vi "GetLCDResultValue.vi"(8 "error in (no error)":errorcluster, 11 "Analysis_LCD_Parameter":T2={"ROI"={"Global Rectangle"=[27, 55, 270, 147], "Contours"=[{"Contour Type"=0, "ROI Type"=3, "Points"=[27, 55, 270, 147]}]}, "Number of Matches Requested"=1} {"Number of Matches Requested" min=1 max=9999}) -> (0 "error out":errorcluster, 3 "ResultValues":string[](array[string]))   [LabVIEW 2015]
uses:
  Controls/LCD/Analysis_LCD_Parameter.ctl
panel:
  in  "data":T1
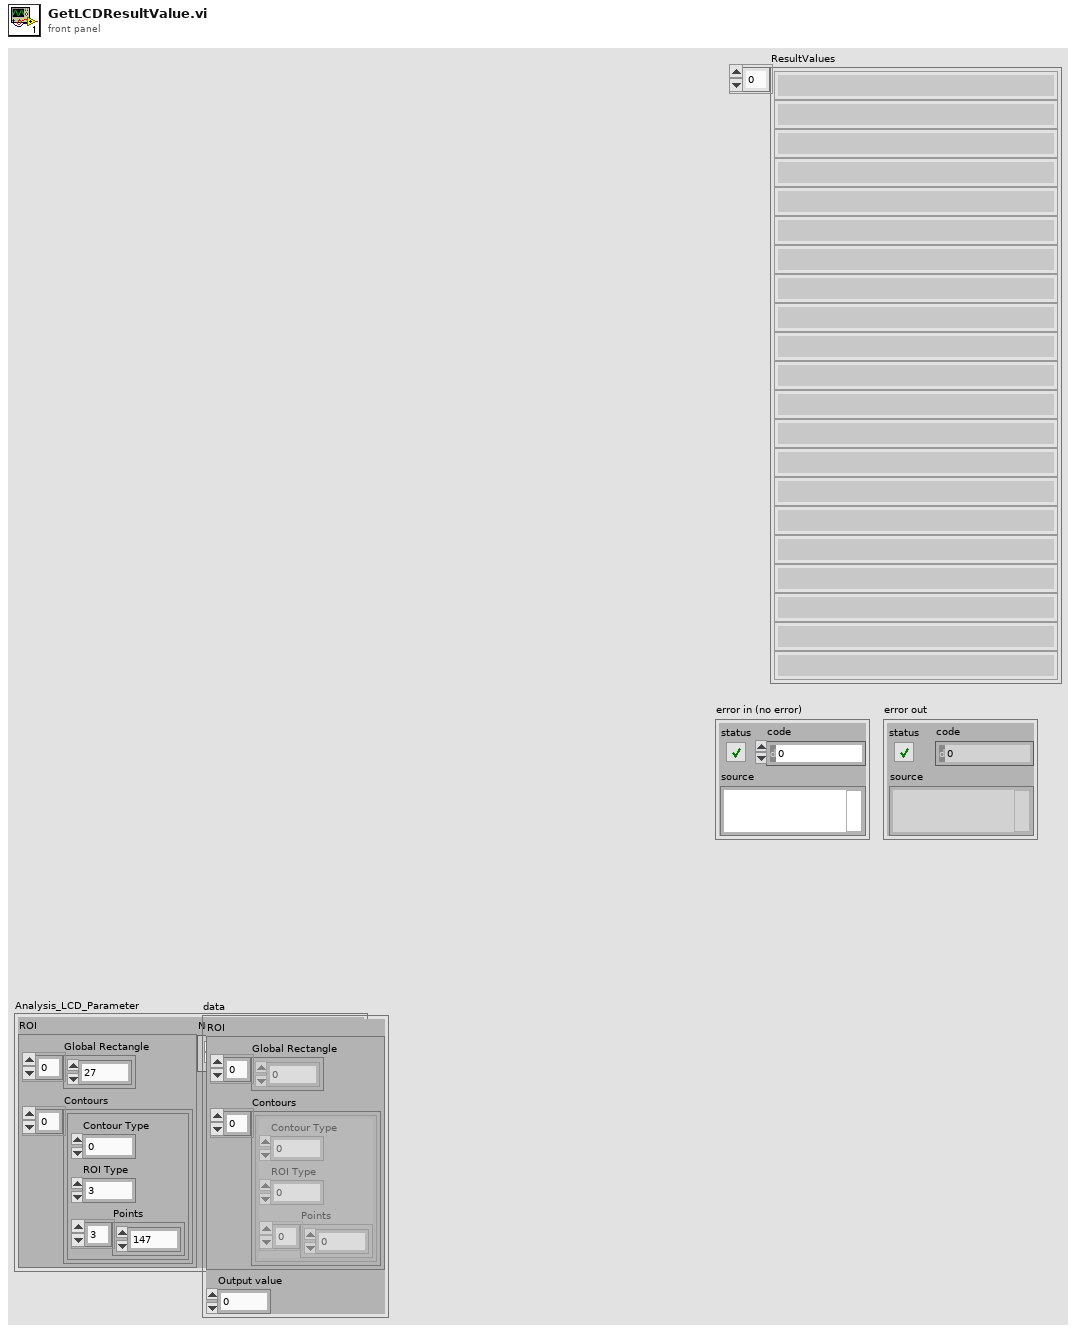
[diagram p1: front panel]
types:
  T1 = cluster{"ROI":cluster{"Global Rectangle":i32[], "Contours":cluster{"Contour Type":u32, "ROI Type":u32, "Points":i32[]}[]}, "Output value":dbl}
  T2 = typedef "Analysis_LCD_Parameter.ctl" = cluster{"ROI":cluster{"Global Rectangle":i32[], "Contours":cluster{"Contour Type":u32, "ROI Type":u32, "Points":i32[]}[]}, "Number of Matches Requested":i32}
  T3 = cluster{"Global Rectangle":i32[], "Contours":cluster{"Contour Type":u32, "ROI Type":u32, "Points":i32[]}[]}
  T4 = cluster{"Contour Type":u32, "ROI Type":u32, "Points":i32[]}[]
  T5 = cluster{"Contour Type":u32, "ROI Type":u32, "Points":i32[]}
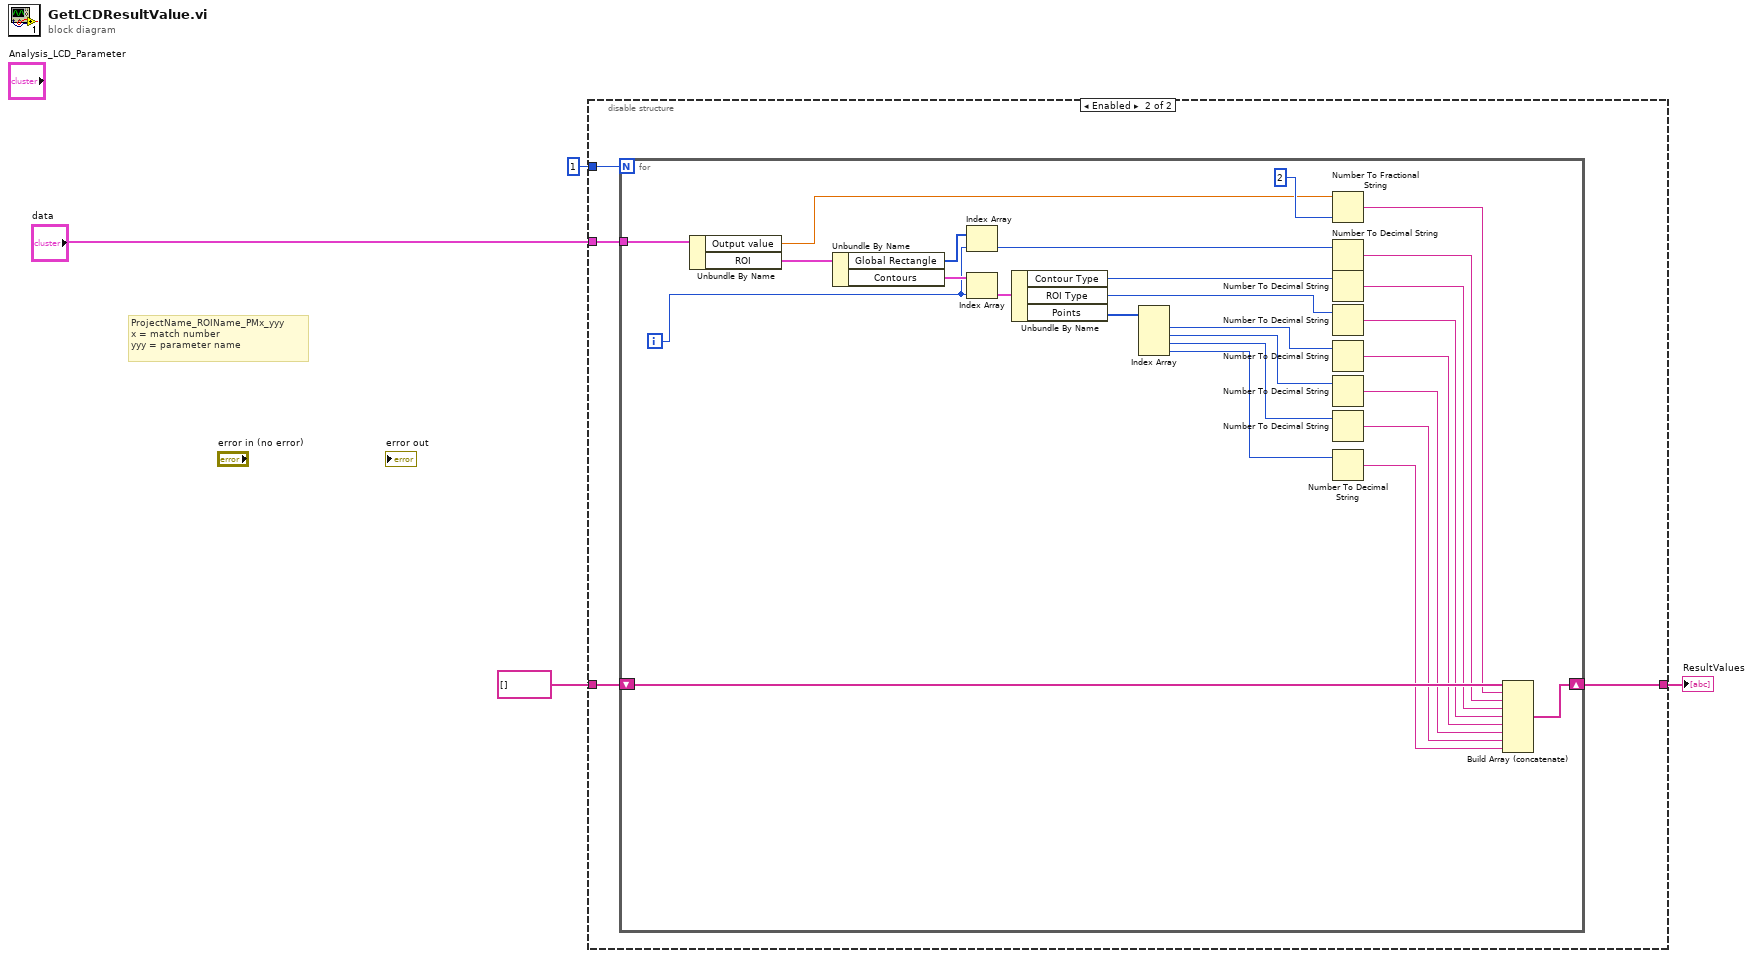
[diagram p0: block diagram]
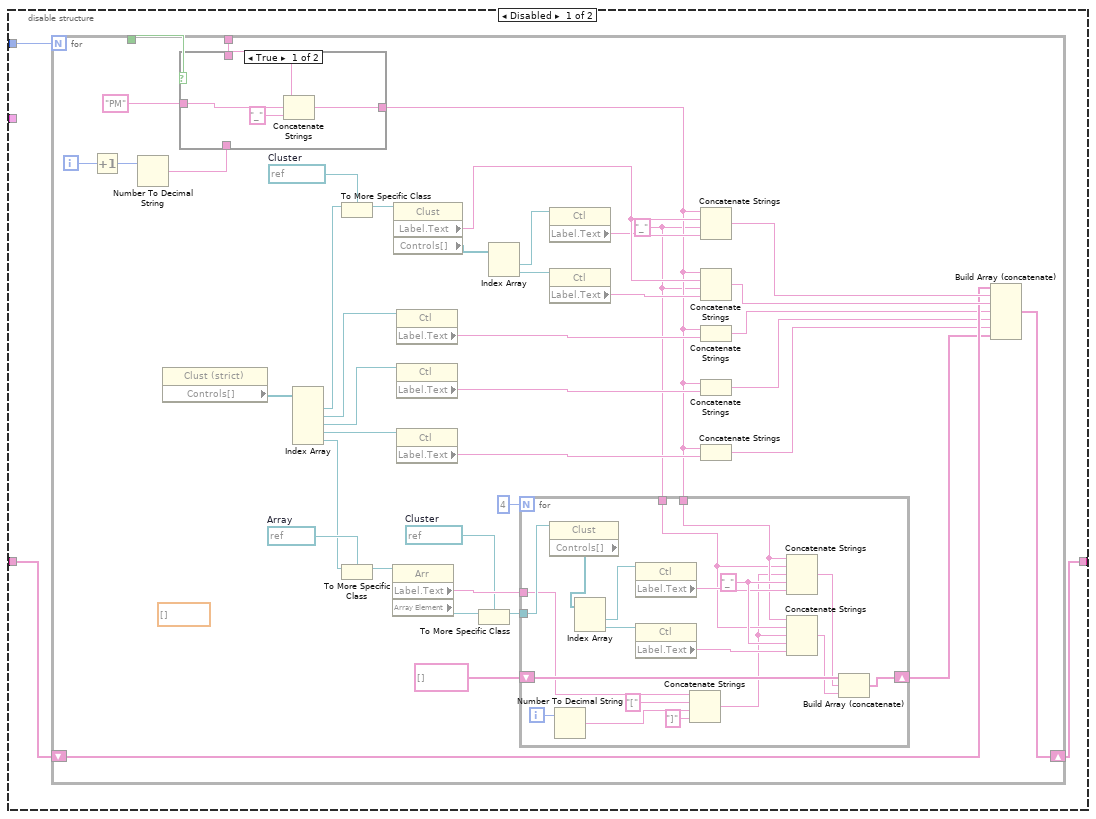
[diagram p2: hidden frame]
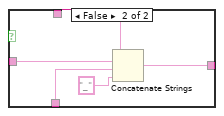
[diagram p3: hidden frame]
diagram:
  # "ProjectName_ROIName_PMx_yyy\nx = match number\nyyy = parameter name"
  n1 = disable-structure shown="Enabled" {
    disable-tunnel: 1 ("Number of Matches Requested") -> [w8 w82]
    disable-tunnel: string[] [] -> [w7 w81]
    disable-tunnel: [w6 w80] -> w3
    disable-tunnel: "data" -> [_ w79]
    frame Disabled {
      n2 = for {
        N: w8 -> [_]
        tunnel: _ -> [w30]
        shift-right: [w32] -> w6
        shift-left: w7 -> [w33]
        tunnel: [w31] -> w5
        i -> [w36]
        w15 = refnum<vi> refnum  # Cluster
        (unwired) dbl[] []
        w20 = refnum<vi> refnum  # Array
        w11 = "_" ("string")
        w46 = refnum<vi> refnum  # Cluster
        n3 = Increment(x=w36) -> (x+1=w35:i32)
        n4 = Number To Decimal String(number=w35) -> (decimal integer string=w29:string)  [unwired: 1 in]
        n5 = property class="Clust (strict)"() -> (reference=w50:refnum<vi>, "Controls[]"=w49:refnum<vi>[])  [unwired: 1 in, 2 out]
        n6 = case shown="True" w31 {
          tunnel: w30 -> [w73 w78]
          tunnel: w29 -> [_ w75]
          tunnel: [w72 w77] -> w12
          tunnel: "PM" ("string") -> [w71 w74]
          frame True {
            n7 = Concatenate Strings(w73, w71, "_" ("string")) -> (w72:string)
          }
          frame False {
            n8 = Concatenate Strings(w78, w74, w75, "_" ("string")) -> (w77:string)
          }
        }
        n9 = Index Array(array=w49) -> (element #1=w48:refnum<vi>, element #2=w27:refnum<vi>, element #3=w26:refnum<vi>, element #4=w39:refnum<vi>, element #5=w19:refnum<vi>)  [unwired: 5 in]
        n10 = To More Specific Class(target class=w46, reference=w48) -> (specific class reference=w47:refnum<vi>)  [unwired: 1 in, 1 out]
        n11 = To More Specific Class(target class=w20, reference=w19) -> (specific class reference=w18:refnum<vi>)  [unwired: 1 in, 1 out]
        n12 = property class="Arr"(reference=w18) -> ("Label.Text"=w17:string, "Array Element"=w14:refnum<vi>)  [unwired: 1 in, 2 out]
        n13 = property class="Clust"(reference=w47) -> ("Label.Text"=w42:string, "Controls[]"=w45:refnum<vi>[])  [unwired: 1 in, 2 out]
        n14 = property class="Ctl"(reference=w27) -> ("Label.Text"=w25:string)  [unwired: 1 in, 2 out]
        n15 = property class="Ctl"(reference=w26) -> ("Label.Text"=w24:string)  [unwired: 1 in, 2 out]
        n16 = property class="Ctl"(reference=w39) -> ("Label.Text"=w34:string)  [unwired: 1 in, 2 out]
        n17 = To More Specific Class(target class=w15, reference=w14) -> (specific class reference=w13:refnum<vi>)  [unwired: 1 in, 1 out]
        n18 = Index Array(array=w45) -> (element #1=w44:refnum<vi>, element #2=w43:refnum<vi>)  [unwired: 2 in]
        n19 = for {
          N: 4 -> [_]
          tunnel: w17 -> [w55]
          tunnel: w13 -> [w69]
          tunnel: w12 -> [w62]
          tunnel: w11 -> [w61]
          shift-right: [w57] -> w9
          shift-left: string[] [] -> [w60]
          i -> [w56]
          w68 = "_" ("string")
          n20 = property class="Clust"(reference=w69) -> ("Controls[]"=w63:refnum<vi>[])  [unwired: 1 in, 2 out]
          n21 = Number To Decimal String(number=w56) -> (decimal integer string=w53:string)  [unwired: 1 in]
          n22 = Index Array(array=w63) -> (element #1=w64:refnum<vi>, element #2=w65:refnum<vi>)  [unwired: 2 in]
          n23 = property class="Ctl"(reference=w64) -> ("Label.Text"=w66:string)  [unwired: 1 in, 2 out]
          n24 = property class="Ctl"(reference=w65) -> ("Label.Text"=w67:string)  [unwired: 1 in, 2 out]
          n25 = Concatenate Strings(w55, "[" ("string"), w53, "]" ("string")) -> (w51:string)
          n26 = Concatenate Strings(w62, w61, w51, w68, w66) -> (w59:string)
          n27 = Concatenate Strings(w62, w61, w51, w68, w67) -> (w58:string)
          n28 = Build Array (concatenate)(w60, w59, w58) -> (w57:string[])
        }
        n29 = property class="Ctl"(reference=w44) -> ("Label.Text"=w41:string)  [unwired: 1 in, 2 out]
        n30 = property class="Ctl"(reference=w43) -> ("Label.Text"=w40:string)  [unwired: 1 in, 2 out]
        n31 = Concatenate Strings(w12, w42, w11, w41) -> (w38:string)
        n32 = Concatenate Strings(w12, w42, w11, w40) -> (w37:string)
        n33 = Concatenate Strings(w12, w25) -> (w21:string)
        n34 = Concatenate Strings(w12, w24) -> (w22:string)
        n35 = Concatenate Strings(w12, w34) -> (w23:string)
        n36 = Build Array (concatenate)(w33, w38, w37, w21, w22, w23, w9) -> (w32:string[])
      }
    }
    frame Enabled {
      n37 = for {
        N: w82 -> [_]
        shift-right: [w106] -> w80
        shift-left: w81 -> [w107]
        tunnel: w79 -> [w108]
        i -> [w99]
        n38 = Unbundle By Name(w108) -> ("Output value"=w104:dbl, "ROI"=w103:T3)
        n39 = Unbundle By Name(w103) -> ("Global Rectangle"=w100:i32[], "Contours"=w102:T4)
        n40 = Index Array(array=w100, index=w99) -> (element=w98:i32)
        n41 = Index Array(array=w102, index=w99) -> (element=w101:T5)
        n42 = Unbundle By Name(w101) -> ("Contour Type"=w97:u32, "ROI Type"=w96:u32, "Points"=w95:i32[])
        n43 = Index Array(array=w95) -> (element #1=w94:i32, element #2=w93:i32, element #3=w92:i32, element #4=w91:i32)  [unwired: 4 in]
        n44 = Number To Fractional String(number=w104, precision (6)=2) -> (F-format string=w90:string)  [unwired: 2 in]
        n45 = Number To Decimal String(number=w98) -> (decimal integer string=w89:string)  [unwired: 1 in]
        n46 = Number To Decimal String(number=w97) -> (decimal integer string=w88:string)  [unwired: 1 in]
        n47 = Number To Decimal String(number=w96) -> (decimal integer string=w87:string)  [unwired: 1 in]
        n48 = Number To Decimal String(number=w94) -> (decimal integer string=w86:string)  [unwired: 1 in]
        n49 = Number To Decimal String(number=w93) -> (decimal integer string=w85:string)  [unwired: 1 in]
        n50 = Number To Decimal String(number=w92) -> (decimal integer string=w84:string)  [unwired: 1 in]
        n51 = Number To Decimal String(number=w91) -> (decimal integer string=w83:string)  [unwired: 1 in]
        n52 = Build Array (concatenate)(w107, w90, w89, w88, w87, w86, w85, w84, w83) -> (w106:string[])
      }
    }
  }
  "ResultValues" <- w3
